vi "dfd_Decide Analysis Resolution (Narrowband).vi"(7 "# freq bins in":i32, 8 "error in (no error)":errorcluster, 11 "narrowband filter in":T1 {"multirate filters"."mMRate_SumWl" min=1 max=32 step=1; "multirate filters"."mMRate_InputIwl" min=1 max=32 step=1; "multirate filters"."mMRate_GainWl" min=1 max=32 step=1; "multirate filters"."mMRate_OutputWl" min=1 max=32 step=1; "multirate filters"."mMRate_InputWl" min=1 max=32 step=1; "multirate filters"."mMRate_CoefWl" min=1 max=32 step=1; "multirate filters"."mMRate_Mode" items=["Default"=-1, "No Rate Change"=0, "Interpolation"=1, "Decimation"=2, "Interpolated"=3, "Rational"=4]}) -> (0 "error out":errorcluster, 3 "narrowband filter out":T1 {"multirate filters"."mMRate_SumWl" min=1 max=32 step=1; "multirate filters"."mMRate_InputIwl" min=1 max=32 step=1; "multirate filters"."mMRate_GainWl" min=1 max=32 step=1; "multirate filters"."mMRate_OutputWl" min=1 max=32 step=1; "multirate filters"."mMRate_InputWl" min=1 max=32 step=1; "multirate filters"."mMRate_CoefWl" min=1 max=32 step=1; "multirate filters"."mMRate_Mode" items=["Default"=-1, "No Rate Change"=0, "Interpolation"=1, "Decimation"=2, "Interpolated"=3, "Rational"=4]}, 5 "# freq bins out":i32)   [LabVIEW 2017, in "NI_DigFilterLicensed.lvlib"]
uses:
  <vilib>/addons/Digital Filter Design/NI_DigFilterLicensed.lvlib
  <vilib>/addons/Digital Filter Design/_Objects.llb/DFD Narrowband Filter Obj.ctl
  <vilib>/addons/Digital Filter Design/_Objects.llb/DFD Multirate Filter Obj.ctl
  <vilib>/addons/Digital Filter Design/_Objects.llb/DFD Multirate Mode.ctl
  <vilib>/addons/Digital Filter Design/_Objects.llb/DFD Coef Norm Type.ctl
  <vilib>/addons/Digital Filter Design/_Objects.llb/DFD Round-off Mode.ctl
  <vilib>/addons/Digital Filter Design/_Objects.llb/DFD FXP MRate Multiply Mode.ctl
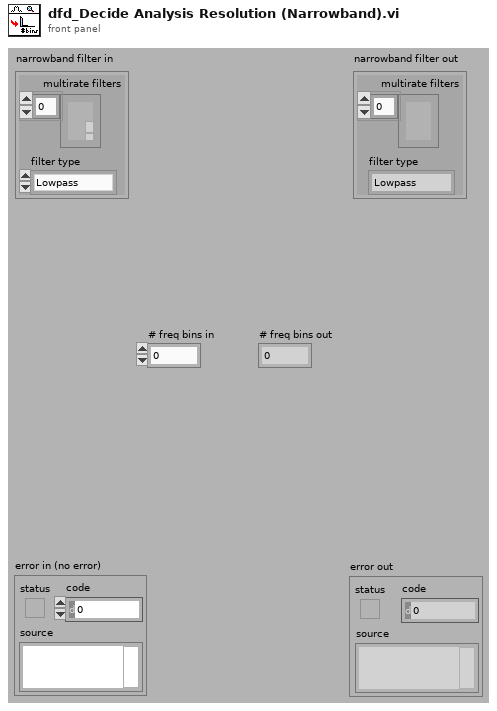
[diagram p1: front panel]
types:
  T1 = typedef "NI_DigFilterLicensed.lvlib/DFD Narrowband Filter Obj.ctl" = cluster{"multirate filters":T2[], "filter type":enum32{"Lowpass", "Highpass", "Bandpass", "Bandstop", "Wideband-Lowpass", "Wideband-Highpass"}}
  T2 = typedef "NI_DigFilterLicensed.lvlib/DFD Multirate Filter Obj.ctl" = cluster{"mMRate_Structure":enum16{"CIC", "FIR", "IIR", "Lattice"}, "mMRate_Mode":T3, "mMRate_Factor":i32, "mMRate_FIRParams":cluster{"mMRate_FIR_H":dbl[], "mMRate_FIR_IsNyquist?":bool, "mMRate_FIR_IsSymmetric?":bool}, "mMRate_CICParams":cluster{"mMRate_CIC_#Stage":i32, "mMRate_CIC_Lag":i32, "mMRate_CIC_Type":enum16{"Lowpass", "Highpass"}}, "mMRate_Order":i32, "mMRate_Version":string, "mMRate_Comments":string, "mMRate_RationalFactor":cluster{"mMRate_L":i32, "mMRate_M":i32}, "mMRate_Fs":dbl, "mMRate_Quantized?":bool, "mMRate_QFilterGain":dbl, "mMRate_CoefWl":i16, "mMRate_Scaling":cluster{"mMRate_ScaleByPowerOf2?":bool, "mMRate_ScaleType":T4}, "mMRate_InputWl":i16, "mMRate_OutputWl":i16, "mMRate_OutputMode":T5, "mMRate_MultMode":T6, "mMRate_BitPruning":bool, "mMRate_GainWl":i16, "mMRate_OutputFwl":i16, "mMRate_SumIwl":i16, "mMRate_InputIwl ":i16, "mMRate_SumWl":i16, "mMRate_CoefIwl":i16}
  T3 = typedef "NI_DigFilterLicensed.lvlib/DFD Multirate Mode.ctl" = i16
  T4 = typedef "NI_DigFilterLicensed.lvlib/DFD Coef Norm Type.ctl" = enum16{"No Norm", "Time Domain 1-Norm", "Time Domain 2-Norm", "Time Domain Inf-Norm"}
  T5 = typedef "NI_DigFilterLicensed.lvlib/DFD Round-off Mode.ctl" = enum16{"Nearest", "Truncation"}
  T6 = typedef "NI_DigFilterLicensed.lvlib/DFD FXP MRate Multiply Mode.ctl" = enum16{"Truncated", "Full"}
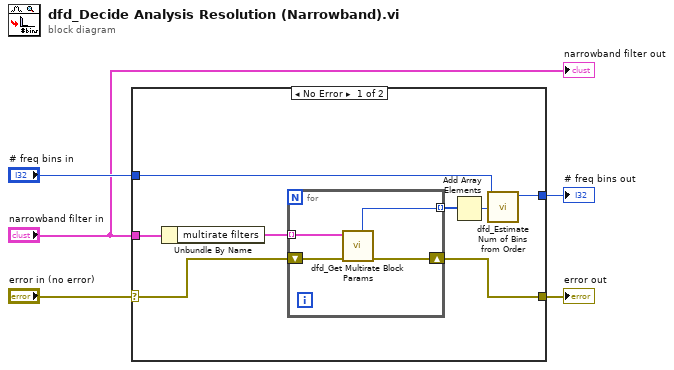
[diagram p0: block diagram]
diagram:
  n1 = case shown="No Error" "error in (no error)" {
    selector: "error in (no error)" -> [w11 w18]
    tunnel: [w10 w18] -> w4
    tunnel: "narrowband filter in" -> [w13 _]
    tunnel: "# freq bins in" -> [w8 _]
    tunnel: [w6 _] -> w2
    frame No Error {
      n2 = Unbundle By Name(w13) -> ("multirate filters"=w12:T2[])
      n3 = for {
        tunnel: w12 -> [w15] mode=indexing
        shift-right: [w17] -> w10
        shift-left: w11 -> [w14]
        tunnel: [w16] -> w9 mode=indexing
        n4 = call <vilib>:"dfd_Get Multirate Block Params.vi"("error in (no error)"=w14, "multirate filter in"=w15) -> ("error out"=w17:errorcluster, "order"=w16:i32)  [unwired: 2 in, 6 out]
      }
      n5 = Add Array Elements(numeric array=w9) -> (sum=w7:i32)
      n6 = call <vilib>:"dfd_Estimate Num of Bins from Order.vi"("order"=w7, "# freq bins in"=w8) -> ("# freq bins out"=w6:i32)  [unwired: 9 out]
    }
    frame Error {
    }
  }
  "# freq bins out" <- w2
  "error out" <- w4
  "narrowband filter out" <- "narrowband filter in"
